vi "LVClass_SlopesPostProcessList GetParameter_Modulator.vi"(0 "SlopesPostProcessorList in":refnum<class "SlopesPostProcessorList.lvclass">, 5 "Position":u32, 11 "error in (no error)":errorcluster) -> (4 "SlopesPostProcessorList out":refnum<class "SlopesPostProcessorList.lvclass">, 8 "filter":T1, 15 "error out":errorcluster)   [LabVIEW 2020, in "SlopesPostProcessorList.lvclass"]
doc: "Get parameters of the Filter processor.\n\n--------------------------------------------------------------------------------\n\n<B>SlopesPostProcessorListIn </B> : SlopesPostProcessorList object.\n<B>SlopesPostProcessorListOut </B> : SlopesPostProcessorList object.\n<B>position </B> : Position of the processor in the SlopesPostProcessorList.\n<B>is_tiltx_filter_on </B> : X tilt filter state.\n<B>is_tilty_filter_on </B> : Y tilt filter state.\n<B>is_curv_filter_on </B> : Curvature filter state.\n<B>is_astig0_filter_on </B> : 0 degree astigmatism filter state.\n<B>is_astig45_filter_on </B> : 45 degree astigmatism filter state.\n<B>is_others_filter_on </B> : All other aberrations filter state.\n<B>ErrorIn </B> : Error\n<B>ErrorOut </B> : Error\n\n--------------------------------------------------------------------------------"
uses:
  SlopesPostProcessorList.lvclass
  SlopesPostProcessorList - Modulator.ctl
  SlopesPostProcessorList.lvclass/SlopesPostProcessorList.ctl
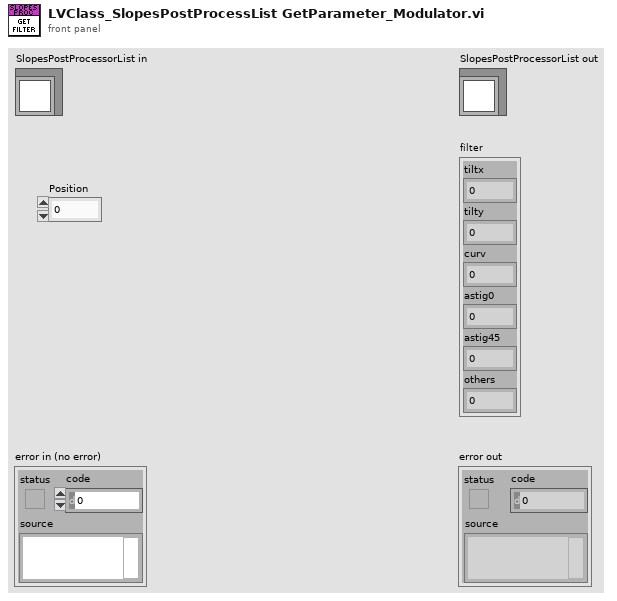
[diagram p1: front panel]
types:
  T1 = typedef "SlopesPostProcessorList - Modulator.ctl" = cluster{"tiltx":sgl, "tilty":sgl, "curv":sgl, "astig0":sgl, "astig45":sgl, "others":sgl}
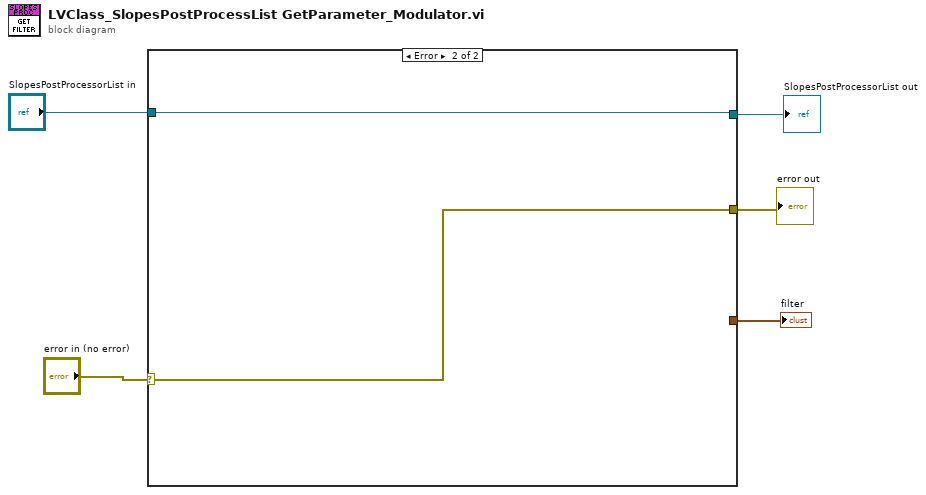
[diagram p0: block diagram]
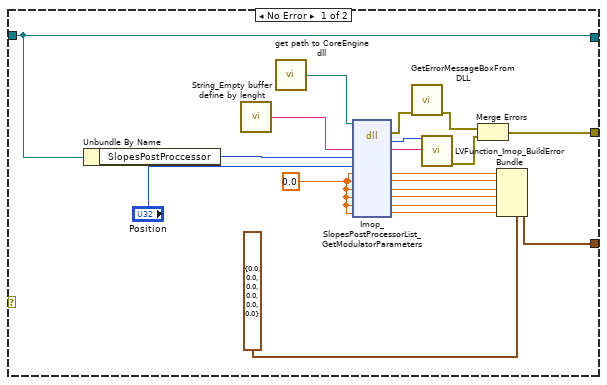
[diagram p2: hidden frame]
diagram:
  n1 = case shown="Error" "error in (no error)" {
    selector: "error in (no error)" -> [_ w26]
    tunnel: "SlopesPostProcessorList in" -> [w20 w27]
    tunnel: [w20 w27] -> w3
    tunnel: [w14 w26] -> w2
    tunnel: [w17 _] -> w1
    frame No Error {
      w13 = sgl 0.0 ("tiltx")
      n2 = Unbundle By Name(w20) -> ("SlopesPostProccessor"=w19:i32)
      n3 = call "String_Empty buffer define by lenght.vi"() -> ("Empty buffer"=w25:string)  [unwired: 1 in]
      n4 = call "get path to CoreEngine dll.vi"() -> ("path to c_interface_vc100.dll"=w22:path)  [unwired: 12 in, 3 out]
      n5 = dll-call lib="D:/soft/HASO_v3/SVN_trunk/ImOpCoreEngine4_LV2011/DLLs/c_interface_vc100.dll" fn="Imop_SlopesPostProcessorList_GetModulatorParameters"(path in=w22, "message"=w25, "objet"=w19, "Position"="Position", "tiltx"=w13, "tilty"=w13, "curv"=w13, "astig0"=w13, "astig45"=w13, "others"=w13) -> (error out=w21:errorcluster, "return type"=w23:i32, "message"=w24:string, "tiltx"=w6:sgl, "tilty"=w7:sgl, "curv"=w8:sgl, "astig0"=w9:sgl, "astig45"=w10:sgl, "others"=w11:sgl)  [unwired: 4 in, 1 out]
      n6 = call "GetErrorMessageBoxFromDLL.vi"("error IN"=w21) -> ("error OUT"=w16:errorcluster)  [unwired: 10 in]
      n7 = call "LVFunction_Imop_BuildError.vi"("code"=w23, "String to Prepend to source (\"\")"=w24) -> ("error out"=w15:errorcluster)  [unwired: 13 in]
      n8 = Merge Errors(w16, w15) -> (w14:errorcluster)
      n9 = Bundle(cluster=T1 {"tiltx"=0.0, "tilty"=0.0, "curv"=0.0, "astig0"=0.0, "astig45"=0.0, "others"=0.0} ("filter"), "tiltx"=w6, "tilty"=w7, "curv"=w8, "astig0"=w9, "astig45"=w10, "others"=w11) -> (w17:T1)
    }
    frame Error {
    }
  }
  "error out" <- w2
  "SlopesPostProcessorList out" <- w3
  "filter" <- w1
